vi "Global_ABORT.vi"() -> ()   [LabVIEW 2015]
panel:
  out "ABORT":bool
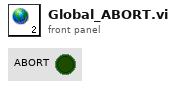
[diagram p1: front panel]
diagram:
